vi "UDP Spark Flag Monitor.vi"(7 "Control Notifier":refnum<notifier>, 8 "error in (no error)":errorcluster, 11 "Spark Status Notifier":refnum<notifier>) -> (0 "error out":errorcluster, 3 "Spark Status Notifier out":refnum<notifier>)   [LabVIEW 2013, in "Breakdown Acoustics Controls.lvlib"]
uses:
  Breakdown Acoustics Controls/Breakdown Acoustics Controls/UDP Heartbeat Globals.vi
  Breakdown Acoustics Controls/Breakdown Acoustics Controls.lvlib
panel:
  out "name":string
  in  "Remote UDP Port":u16=31416
  out "Spark Flag Synch\nLoop Time (ms)":u32
  out "Spark!":bool
  in  "Local UDP Port":u16=31417
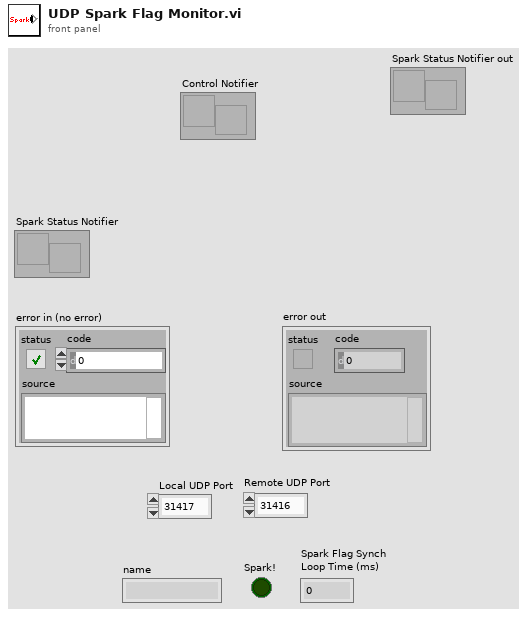
[diagram p1: front panel]
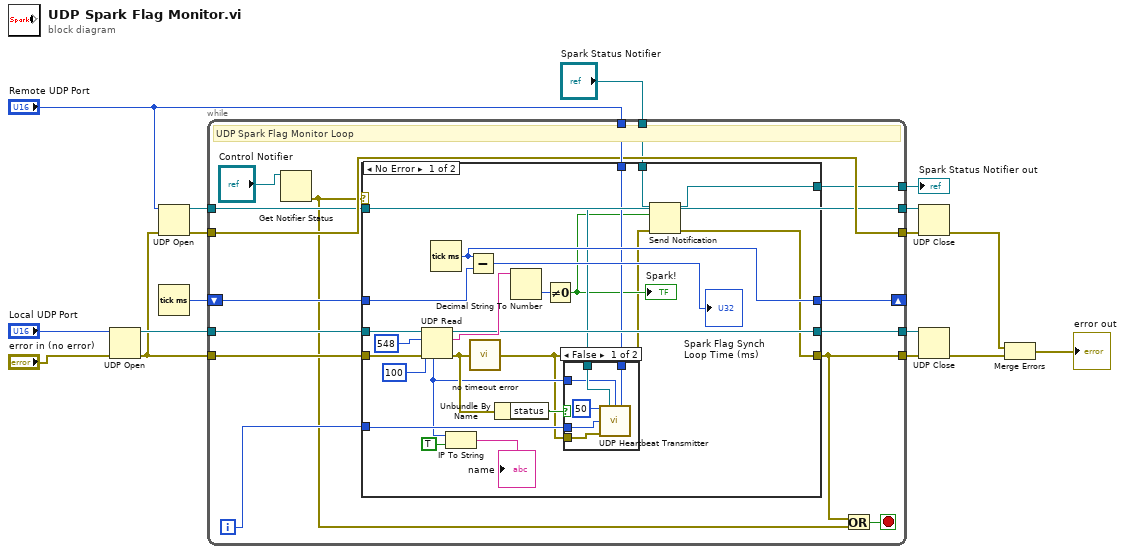
[diagram p0: block diagram]
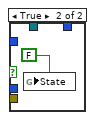
[diagram p2: hidden frame]
diagram:
  n1 = UDP Open(8:"error in (no error)", 11:"Local UDP Port") -> (port=w16:refnum<k16>, 0:w10:errorcluster)  [unwired: 3 in, 1 out]
  n2 = UDP Open(8:w10, 11:"Remote UDP Port") -> (port=w11:refnum<k16>, 0:w9:errorcluster)  [unwired: 3 in, 1 out]
  n3 = Tick Count (ms)() -> (millisecond timer value=w13:u32)
  n4 = while {
    tunnel: w16 -> [w32]
    tunnel: w10 -> [w31]
    tunnel: [w22] -> w15
    tunnel: [w26] -> w14
    shift-right: [w28] -> _
    shift-left: w13 -> [w29]
    tunnel: "Remote UDP Port" -> [w25]
    tunnel: w11 -> [w23]
    tunnel: [w24] -> w8
    tunnel: w9 -> [w24]
    tunnel: [w23] -> w7
    tunnel: "Spark Status Notifier" -> [w19]
    tunnel: [w18] -> w1
    i -> [w27]
    stop <- w30 stop-if-true
    # "UDP Spark Flag Monitor Loop"
    n5 = Get Notifier Status(notifier="Control Notifier") -> (error out=w20:errorcluster)  [unwired: 1 in, 4 out]
    n6 = case shown="No Error" w20 {
      tunnel: w32 -> [w54 w65]
      tunnel: w31 -> [w53 w64]
      tunnel: w29 -> [w50 w66]
      tunnel: [w48 w66] -> w28
      tunnel: w27 -> [w45 _]
      tunnel: [w43 w65] -> w26
      tunnel: w25 -> [w42 _]
      tunnel: w23 -> [w41 _]
      tunnel: [w34 w64] -> w22
      tunnel: w19 -> [w37 w63]
      tunnel: [w33 w63] -> w18
      frame No Error {
        n7 = UDP Read(connection ID=w54, max size (548)=548 ("max bytes/read"), timeout ms (25000)=100, 8:w53) -> (data out=w55:string, error out=w46:errorcluster, 3:w43:refnum<k16>, 6:w40:u32)  [unwired: 1 out]
        n8 = Tick Count (ms)() -> (millisecond timer value=w48:u32)
        n9 = IP To String(1:TRUE ("dot notation? (F)"), 2:w40) -> (0:→"name":string)
        n10 = Subtract(x=w48, y=w50) -> (x-y=→"Spark Flag Synch\nLoop Time (ms)":u32)
        n11 = call "no timeout error.vi"("error in (no error)"=w46) -> ("error out"=w35:errorcluster)
        n12 = Unbundle By Name(w46) -> ("status"=w44:bool)
        n13 = Decimal String To Number(string=w55) -> (number=w51:i32)  [unwired: 2 in, 1 out]
        n14 = Not Equal To 0?(x=w51) -> (x != 0?=w36:bool)
        "Spark!" <- w36
        n15 = case shown="False" w44 {
          tunnel: w45 -> [w60 _]
          tunnel: w35 -> [w59 _]
          tunnel: w41 -> [w58 _]
          tunnel: w42 -> [w57 _]
          tunnel: w40 -> [w56 _]
          frame False {
            n16 = call "UDP Heartbeat Transmitter.vi"("Interval Length"=50, "connection ID"=w58, "Remote UDP Address"=w56, "Remote UDP Port"=w57, "Count"=w60, "error in (no error)"=w59) -> ()  [unwired: 9 in, 1 out]
          }
          frame True {
            n17 = global write "UDP Heartbeat Globals.vi" "State"(FALSE) -> ()
          }
        }
        n18 = Send Notification(notification=w36, notifier=w37, error in (no error)=w35) -> (notifier out=w33:refnum<notifier>, error out=w34:errorcluster)
      }
      frame Error {
      }
    }
    n19 = Or(x=w22, y=w20) -> (x .or. y?=w30:bool)
  }
  "Spark Status Notifier out" <- w1
  n20 = UDP Close(connection ID=w7, 8:w8) -> (error out=w6:errorcluster)  [unwired: 1 out]
  n21 = UDP Close(connection ID=w14, 8:w15) -> (error out=w5:errorcluster)  [unwired: 1 out]
  n22 = Merge Errors(w6, w5) -> (→"error out":errorcluster)
